vi "RTM - Export to XML.vi"(8 "error in (no error)":errorcluster, 11 "Node Ptr":u64 format="%.0x") -> (0 "error out":errorcluster)   [LabVIEW 2016, in "UDP-Custom-Device System Explorer.lvlib"]
uses:
  UDP-Custom-Device System Explorer.lvlib
  <vilib>/NI VeriStand/Custom Device Tools/Custom Device Utility Library/Custom Device Utility Library.lvlib
panel:
  in  "Tag":string
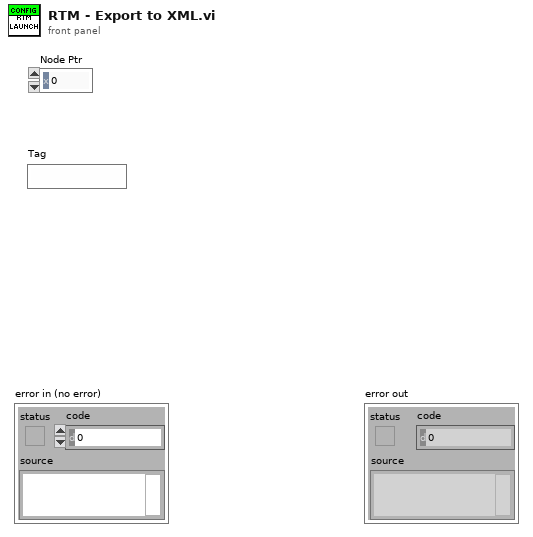
[diagram p1: front panel]
types:
  T1 = typedef "Custom Device API.lvlib/Custom Device Item Ref.ctl" = u64
  T2 = typedef "UDP-Custom-Device System Explorer.lvlib/XML - Header Data.ctl" = cluster{"Revision (\"Major.Minor.Fix.Build\")":string, "Creation Date (\"yyyy-mm-dd\")":string, "Controller Name":string}
  T3 = typedef "UDP-Custom-Device System Explorer.lvlib/XML - Group.ctl" = cluster{"Freq":i32, "Tx Channels":T4[], "Rx Channels":T4[]}
  T4 = typedef "UDP-Custom-Device System Explorer.lvlib/XML - Channel.ctl" = cluster{"Channel Name":string, "Data Type":u16, "Description":string, "Unit":string}
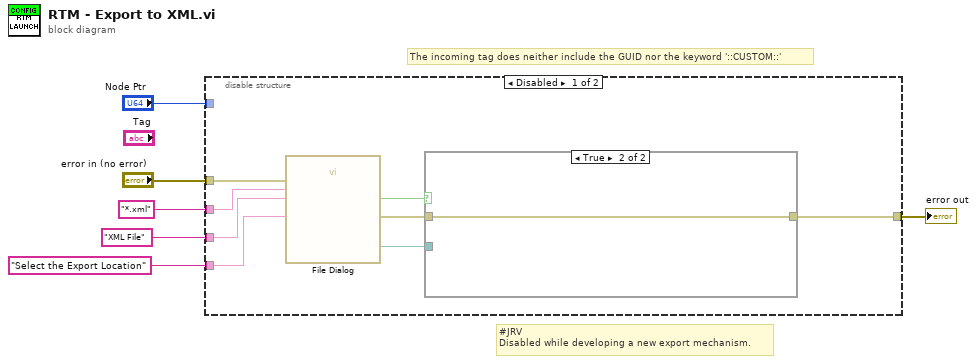
[diagram p0: block diagram]
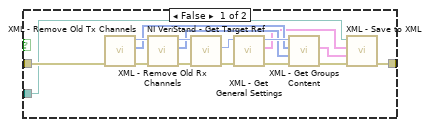
[diagram p2: hidden frame]
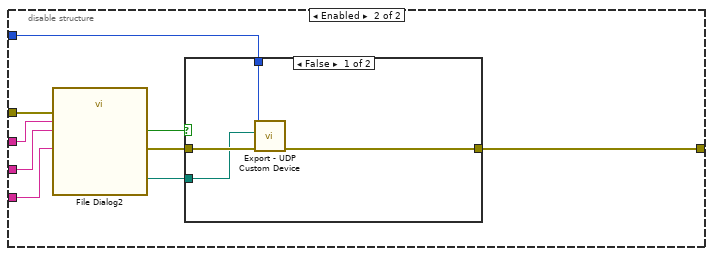
[diagram p3: hidden frame]
diagram:
  # "#JRV\nDisabled while developing a new export mechanism."
  # "The incoming tag does neither include the GUID nor the keyword '::CUSTOM::'"
  n1 = disable-structure shown="Disabled" {
    disable-tunnel: "*.xml" ("pattern (all files)") -> [w14 w38]
    disable-tunnel: "XML File" ("pattern label") -> [w13 w37]
    disable-tunnel: "Select the Export Location" ("prompt") -> [w12 w36]
    disable-tunnel: "error in (no error)" -> [w11 w35]
    disable-tunnel: [w7 w39] -> w2
    disable-tunnel: "Node Ptr" -> [_ w40]
    frame Disabled {
      n2 = call "File Dialog"("prompt"=w12, "error in"=w11, "pattern (all files)"=w14, "pattern label"=w13) -> ("selected path"=w8:path, "cancelled"=w10:bool, "error out"=w9:errorcluster)  [unwired: 8 in, 1 out]
      n3 = case shown="True" w10 {
        tunnel: w9 -> [w25 w31]
        tunnel: w8 -> [w22 _]
        tunnel: [w15 w31] -> w7
        frame False {
          n4 = call "XML - Remove Old Tx Channels.vi"("error in (no error)"=w25) -> ("error out"=w26:errorcluster, "Tx Dependent Refs"=w21:T1[], "Device Item Ref out"=w24:T1)  [unwired: 8 in]
          n5 = call "XML - Remove Old Rx Channels.vi"("error in (no error)"=w26, "Device Item Ref in"=w24) -> ("error out"=w19:errorcluster, "Rx Dependent Refs"=w20:T1[], "Device Item Ref out"=w23:T1)  [unwired: 7 in]
          n6 = call <vilib>:"NI VeriStand - Get Target Ref.vi"("error in"=w19, "Item Ref in"=w23) -> ("error out"=w29:errorcluster, "Target Ref"=w28:T1)  [unwired: 6 in, 2 out]
          n7 = call "XML - Get General Settings.vi"("error in (no error)"=w29, "Target Ref in"=w28) -> ("error out"=w30:errorcluster, "XML Header Data"=w18:T2, "Target Ref out"=w27:T1)  [unwired: 7 in]
          n8 = call "XML - Get Groups Content.vi"("error in (no error)"=w30, "Rx"=w20, "Tx"=w21, "Target Ref In"=w27) -> ("error IO"=w16:errorcluster, "Groups"=w17:T3[])  [unwired: 5 in, 1 out]
          n9 = call "XML - Save to XML.vi"("error in"=w16, "Channel Groups"=w17, "XML Header Data"=w18, "XML File Path"=w22) -> ("error out"=w15:errorcluster)  [unwired: 7 in]
        }
        frame True {
        }
      }
    }
    frame Enabled {
      n10 = call "File Dialog2"("prompt"=w36, "error in"=w35, "pattern (all files)"=w38, "pattern label"=w37) -> ("selected path"=w33:path, "cancelled"=w32:bool, "error out"=w34:errorcluster)  [unwired: 8 in, 1 out]
      n11 = case shown="False" w32 {
        tunnel: w40 -> [w44 _]
        tunnel: [w43 w45] -> w39
        tunnel: w34 -> [w42 w45]
        tunnel: w33 -> [w41 _]
        frame False {
          n12 = call "Export - UDP Custom Device.vi"("error in (no error)"=w42, "Target File"=w41, "Device Item Ref in"=w44) -> ("error out"=w43:errorcluster)  [unwired: 8 in]
        }
        frame True {
        }
      }
    }
  }
  "error out" <- w2
